vi "Read Forces in Stiffness Summary.vi"(11 "StiffnessCalculator in":refnum<class "StiffnessCalculator.lvclass">) -> (2 "Forces in Stiffness Summary":dbl[unit][](array[numeric]) min=-888.0 max=888.0, 3 "StiffnessCalculator out":refnum<class "StiffnessCalculator.lvclass">)   [LabVIEW 2015, in "StiffnessCalculator.lvclass"]
uses:
  StiffnessCalculator.lvclass
  StiffnessCalculator.lvclass/StiffnessCalculator.ctl
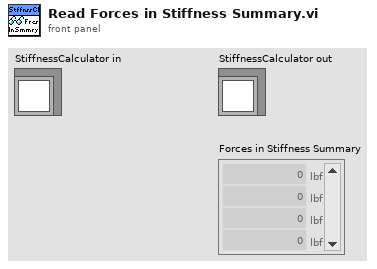
[diagram p1: front panel]
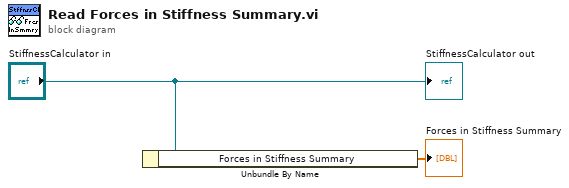
[diagram p0: block diagram]
diagram:
  n1 = Unbundle By Name("StiffnessCalculator in") -> ("Forces in Stiffness Summary"=→"Forces in Stiffness Summary":dbl[unit][])
  "StiffnessCalculator out" <- "StiffnessCalculator in"
